vi "Capture Single Image.vi"(7 "calRefPath":string, 8 "error in (no error)":errorcluster, 9 "nMode":u32, 10 "pImage":u16[](array[numeric]), 11 "nSensorIP":u32) -> (0 "error out":errorcluster, 2 "pImage out":u16[](array[numeric]), 3 "function return":i32)   [LabVIEW 2017, in "BonTechWrapperLibrary.lvlib"]
doc: "extern \"C\" BONTECHLIBRARY_API int __stdcall CaptureSingleImage(unsigned int nSensorIP);\n\nextern \"C\" BONTECHLIBRARY_API int __stdcall CaptureSingleImage(unsigned int nSensorIP, unsigned short* pImage, unsigned int nMode, LPCTSTR calRefPath);"
uses:
  BonTechWrapperLibrary.lvlib
  BonTechWrapperLibrary.dll
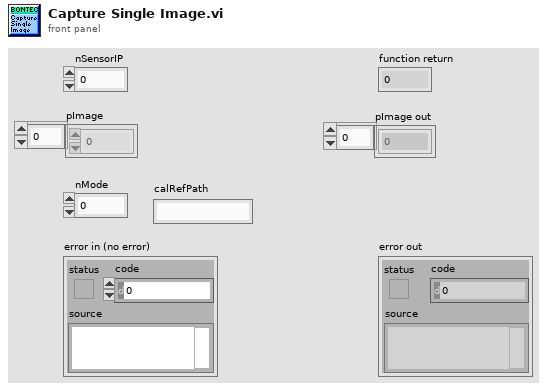
[diagram p1: front panel]
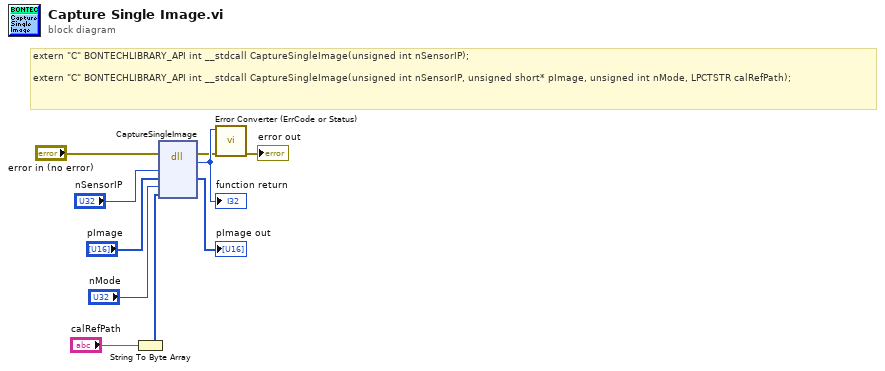
[diagram p0: block diagram]
diagram:
  # "extern \"C\" BONTECHLIBRARY_API int __stdcall CaptureSingleImage(unsigned int nSensorIP);\n\nextern \"C\" BONTECHLIBRARY_API int __stdcall CaptureSingleImage(unsigned int nSensorIP, unsigned short* pImage, unsigned int nMode, LPCTSTR calRefPath);"
  n1 = String To Byte Array(string="calRefPath") -> (unsigned byte array=w1:u8[])
  n2 = dll-call lib="C:/Users/Achuthaperumal/SourceCodes/BonTechWrapperLibrary/BonTechWrapperLibrary/x64/Release/BonTechWrapperLibrary.*" fn="CaptureSingleImage"(error in="error in (no error)", "nSensorIP"="nSensorIP", "pImage"="pImage", "nMode"="nMode", "calRefPath"=w1) -> (error out=w3:errorcluster, "return type"=w10:i32, "pImage"=→"pImage out":u16[])  [unwired: 5 in, 1 out]
  "function return" <- w10
  n3 = call "Error Converter (ErrCode or Status).vi"("error in (no error)"=w3, "error code"=w10) -> ("error out"=→"error out":errorcluster)  [unwired: 9 in]
